vi "BlackBodyFurnace Visualization.vi"() -> ()   [LabVIEW 2018]
panel:
  in  "DAQmx Device Name":tag
  out "element":cluster{dbl[], dbl[]}
  out "XY Graph 3":cluster{dbl[], dbl[]}(graph)
  out "XY Graph 2":cluster{dbl[], dbl[]}(graph)
  in  "Reset":bool=TRUE
  out "XY Graph":cluster{"Y":dbl[], "Y":dbl[]}[](graph)
  in  "stop":bool
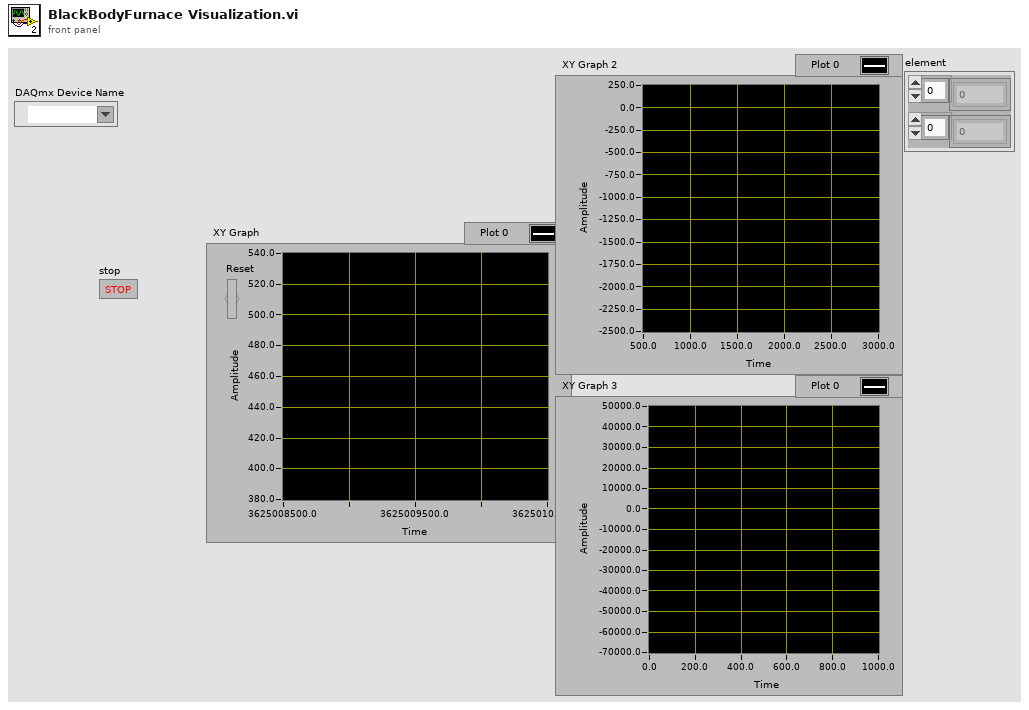
[diagram p1: front panel]
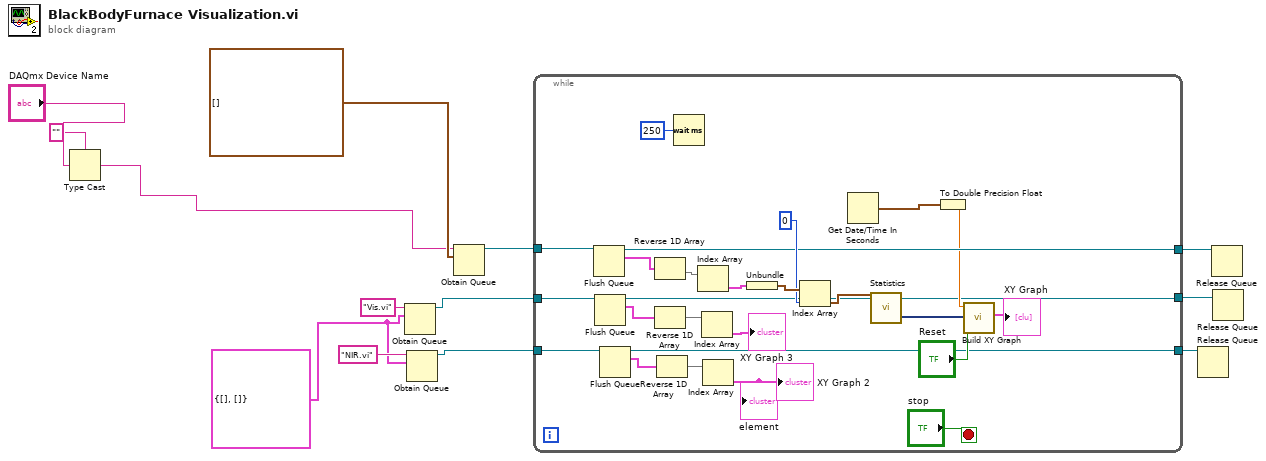
[diagram p0: block diagram]
diagram:
  w4 = cluster{dbl[], dbl[]} {[], []}
  n1 = Type Cast(type="", x="DAQmx Device Name") -> (*(type *) &x=w2:string)
  n2 = Obtain Queue(name (unnamed)="Vis.vi", element data type=w4) -> (queue out=w8:refnum<queue>)  [unwired: 3 in, 2 out]
  n3 = Obtain Queue(name (unnamed)="NIR.vi", element data type=w4) -> (queue out=w7:refnum<queue>)  [unwired: 3 in, 2 out]
  n4 = Obtain Queue(name (unnamed)=w2, element data type=waveform(dbl)[] [] ("data")) -> (queue out=w12:refnum<queue>)  [unwired: 3 in, 2 out]
  n5 = while {
    tunnel: w12 -> [w38]
    tunnel: [w32] -> w11
    tunnel: w8 -> [w23]
    tunnel: w7 -> [w22]
    tunnel: [w17] -> w6
    tunnel: [w16] -> w5
    stop <- "stop" stop-if-true
    n6 = Flush Queue(queue=w38) -> (queue out=w32:refnum<queue>, remaining elements=w37:cluster{"data":waveform(dbl)[]}[])  [unwired: 1 in, 1 out]
    n7 = Flush Queue(queue=w23) -> (queue out=w17:refnum<queue>, remaining elements=w20:cluster{dbl[], dbl[]}[])  [unwired: 1 in, 1 out]
    n8 = Flush Queue(queue=w22) -> (queue out=w16:refnum<queue>, remaining elements=w21:cluster{dbl[], dbl[]}[])  [unwired: 1 in, 1 out]
    n9 = Reverse 1D Array(array=w37) -> (reversed array=w36:cluster{"data":waveform(dbl)[]}[])
    n10 = Reverse 1D Array(array=w20) -> (reversed array=w18:cluster{dbl[], dbl[]}[])
    n11 = Reverse 1D Array(array=w21) -> (reversed array=w19:cluster{dbl[], dbl[]}[])
    n12 = Wait (ms)(milliseconds to wait=u32 250) -> ()  [unwired: 1 out]
    n13 = Index Array(array=w36) -> (element=w35:cluster{"data":waveform(dbl)[]})  [unwired: 1 in]
    n14 = Index Array(array=w18) -> (element=→"XY Graph 3":cluster{dbl[], dbl[]})  [unwired: 1 in]
    n15 = Index Array(array=w19) -> (element=→"XY Graph 2" →"element":cluster{dbl[], dbl[]})  [unwired: 1 in]
    n16 = Unbundle(w35) -> ("data"=w34:waveform(dbl)[])
    n17 = Index Array(array=w34, index=0) -> (element=w29:waveform(dbl))
    n18 = Get Date/Time In Seconds() -> (seconds since 1Jan1904=w26:timestamp)
    n19 = call "Statistics"("Signals"=w29) -> ("Arithmetic Mean"=w27:dynamicdata)  [unwired: 25 in, 1 out]
    n20 = To Double Precision Float(number=w26) -> (double precision float=w25:dbl)
    n21 = call "Build XY Graph"("Reset"="Reset", "Y Input"=w27, "X Input"=w25) -> ("XY Graph"=→"XY Graph":cluster{"X":dbl[], "Y":dbl[]}[])  [unwired: 7 in, 1 out]
  }
  n22 = Release Queue(queue=w5) -> ()  [unwired: 2 in, 3 out]
  n23 = Release Queue(queue=w11) -> ()  [unwired: 2 in, 3 out]
  n24 = Release Queue(queue=w6) -> ()  [unwired: 2 in, 3 out]
